vi "Close 3458A.vi"(8 "error in (no error)":errorcluster, 9 "keep display in whatever mode? (False)":bool, 10 "Reset to preset mode (True)":bool=TRUE, 11 "VISA resource name":refnum<visa-resource-name>) -> (0 "error out":errorcluster)   [LabVIEW 2020, in "3458A Virtual Digitizer.lvlib" / "3458A Digitizing Low Levels.lvlib"]
doc: "Performs an instrument error query before terminating the software connection to the instrument. Always goes to loacal mode. Optinally resets instrument to default mode.\n\nNote: Reentrant VI so it can be executed in parallel for multiple 3458A sessions."
uses:
  3458A Digitizing Low Levels.lvlib
  3458A Basic Driver/3458A Basic Driver.lvlib
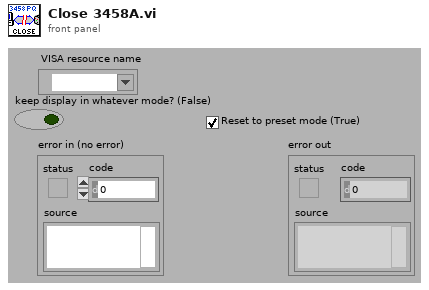
[diagram p1: front panel]
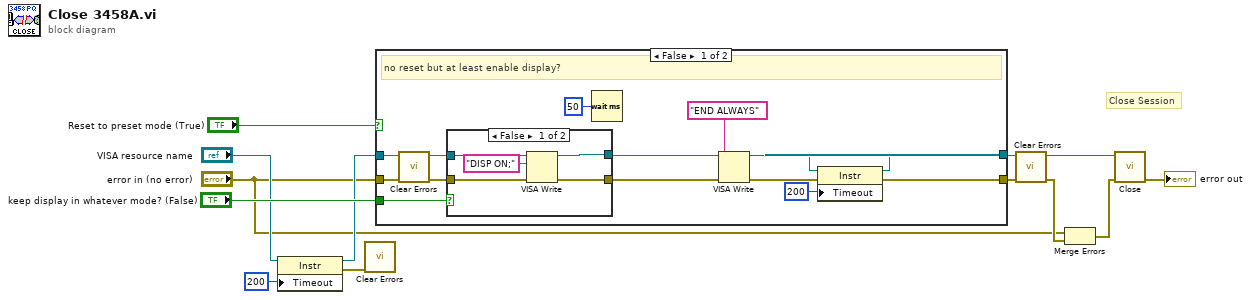
[diagram p0: block diagram]
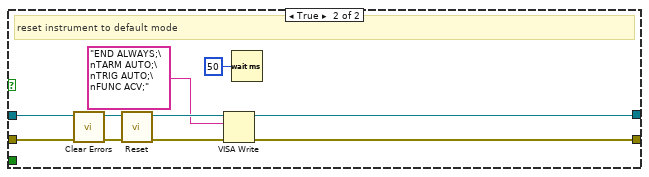
[diagram p3: hidden frame]
diagram:
  # "Close Session"
  n1 = property class="Instr"(reference="VISA resource name", "Timeout"=u32 200 ("General Settings:Timeout Value")) -> (reference out=w4:refnum<visa-resource-name>, error out=w2:errorcluster)  [unwired: 1 in]
  n2 = call <vilib>:"Clear Errors.vi"("error in (no error)"=w2) -> ()  [unwired: 5 in, 2 out]
  n3 = case shown="False" "Reset to preset mode (True)" {
    tunnel: "error in (no error)" -> [w24 w41]
    tunnel: w4 -> [w25 w39]
    tunnel: [w18 w36] -> w8
    tunnel: [w16 w35] -> w7
    tunnel: "keep display in whatever mode? (False)" -> [w22 _]
    frame False {
      # "no reset but at least enable display?"
      n4 = call <vilib>:"Clear Errors.vi"("error in (no error)"=w24) -> ("error out"=w19:errorcluster)  [unwired: 5 in, 1 out]
      n5 = case shown="False" w22 {
        tunnel: [w30 w31] -> w14
        tunnel: [w29 w32] -> w13
        tunnel: w25 -> [w28 w32]
        tunnel: w19 -> [w27 w31]
        frame False {
          n6 = VISA Write(VISA resource name=w28, write buffer="DISP ON;", error in (no error)=w27) -> (VISA resource name out=w29:refnum<visa-resource-name>, error out=w30:errorcluster)  [unwired: 1 out]
        }
        frame True {
        }
      }
      n7 = Wait (ms)(milliseconds to wait=u32 50) -> ()  [unwired: 1 out]
      n8 = VISA Write(VISA resource name=w13, write buffer="END ALWAYS", error in (no error)=w14) -> (VISA resource name out=w17:refnum<visa-resource-name>, error out=w21:errorcluster)  [unwired: 1 out]
      n9 = property class="Instr"(reference=w17, error in=w21, "Timeout"=u32 200 ("General Settings:Timeout Value")) -> (reference out=w16:refnum<visa-resource-name>, error out=w18:errorcluster)
    }
    frame True {
      # "reset instrument to default mode"
      n10 = call <vilib>:"Clear Errors.vi"("error in (no error)"=w41) -> ("error out"=w40:errorcluster)  [unwired: 5 in, 1 out]
      n11 = call "Reset.vi"("error in (no error)"=w40, "VISA resource name"=w39) -> ("error out"=w38:errorcluster, "VISA resource name out"=w37:refnum<visa-resource-name>)  [unwired: 8 in]
      n12 = VISA Write(VISA resource name=w37, write buffer="END ALWAYS;\nTARM AUTO;\nTRIG AUTO;\nFUNC ACV;", error in (no error)=w38) -> (VISA resource name out=w35:refnum<visa-resource-name>, error out=w36:errorcluster)  [unwired: 1 out]
      n13 = Wait (ms)(milliseconds to wait=u32 50) -> ()  [unwired: 1 out]
    }
  }
  n14 = call <vilib>:"Clear Errors.vi"("error in (no error)"=w8) -> ("error out"=w11:errorcluster)  [unwired: 5 in, 1 out]
  n15 = Merge Errors("error in (no error)", w11) -> (w10:errorcluster)
  n16 = call "Close.vi"("error in (no error)"=w10, "VISA resource name"=w7) -> ("error out"=→"error out":errorcluster)  [unwired: 9 in]
